vi "insertBundleUnbundle.vi"(2 "error in (no error)":errorcluster, 3 "Controls Cluster":T1(array[cluster]), 4 "action vi path":path) -> (0 "error out":errorcluster, 1 "Indicators":cluster{"Style":u32, "Label.Text":string, i32}[](array[cluster]))   [LabVIEW 2009, in "HGF_VisitorGenerator.lvlib"]
doc: "insert bundle and unbundle node to visitors action.vi"
uses:
  HGF_VisitorGenerator.lvlib
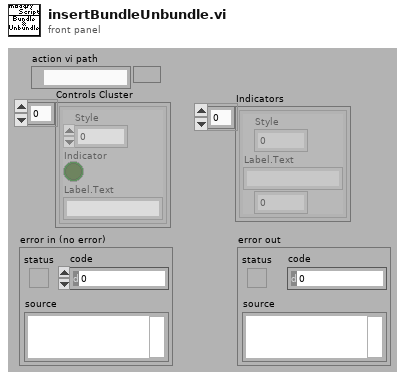
[diagram p1: front panel]
types:
  T1 = cluster{"Style":u32, "Indicator":bool, "Label.Text":string}[]
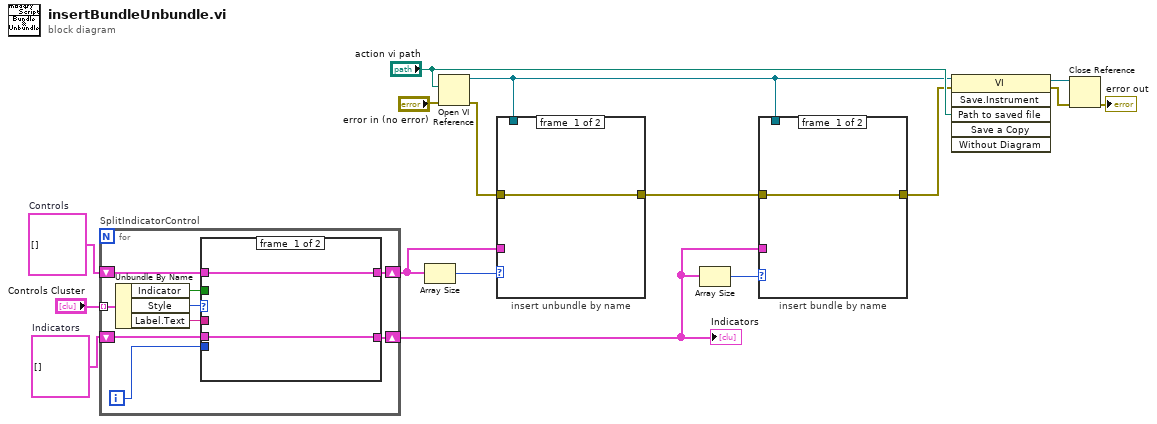
[diagram p0: block diagram]
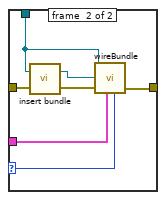
[diagram p2: hidden frame]
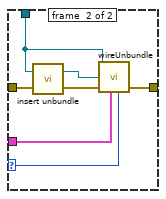
[diagram p3: hidden frame]
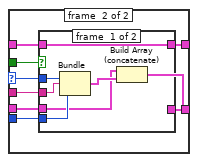
[diagram p4: hidden frame]
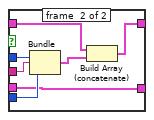
[diagram p5: hidden frame]
diagram:
  w16 = cluster{"Style":u32, "Label.Text":string, i32}[] []  # Indicators
  w15 = cluster{"Style":u32, "Label.Text":string, i32}[] []  # Controls
  n1 = for "SplitIndicatorControl" {
    tunnel: "Controls Cluster" -> [w25] mode=indexing
    shift-right: [w19] -> w2
    shift-left: w15 -> [w21]
    shift-right: [w17] -> w7
    shift-left: w16 -> [w18]
    i -> [w20]
    n2 = Unbundle By Name(w25) -> ("Indicator"=w23:bool, "Style"=w24:u32, "Label.Text"=w22:string)
    n3 = case shown="0" w24 {
      selector: w24 -> [_ w34]
      tunnel: w23 -> [_ w35]
      tunnel: w22 -> [_ w33]
      tunnel: w21 -> [w27 w31]
      tunnel: w20 -> [_ w32]
      tunnel: [w27 w30] -> w19
      tunnel: w18 -> [w26 w29]
      tunnel: [w26 w28] -> w17
      frame #0 {
      }
      frame #1 {
        n4 = case shown="False" w35 {
          tunnel: w34 -> [w42 w47]
          tunnel: w33 -> [w41 w46]
          tunnel: w32 -> [w40 w45]
          tunnel: w31 -> [w38 w49]
          tunnel: [w38 w48] -> w30
          tunnel: w29 -> [w37 w43]
          tunnel: [w36 w43] -> w28
          frame #0 {
            n5 = Bundle("Style"=w42, "Label.Text"=w41, w40) -> (w39:cluster{"Style":u32, "Label.Text":string, i32})  [unwired: 1 in]
            n6 = Build Array (concatenate)(w37, w39) -> (w36:cluster{"Style":u32, "Label.Text":string, i32}[])
          }
          frame #1 {
            n7 = Bundle("Style"=w47, "Label.Text"=w46, w45) -> (w44:cluster{"Style":u32, "Label.Text":string, i32})  [unwired: 1 in]
            n8 = Build Array (concatenate)(w49, w44) -> (w48:cluster{"Style":u32, "Label.Text":string, i32}[])
          }
        }
      }
    }
  }
  "Indicators" <- w7
  n9 = Array Size(array=w2) -> (size(s)=w1:i32)
  n10 = Open VI Reference(vi path="action vi path", error in (no error)="error in (no error)") -> (vi reference=w5:refnum<vi>, error out=w12:errorcluster)  [unwired: 4 in]
  n11 = case "insert unbundle by name" shown="Default" w1 {
    selector: w1 -> [_ w52]
    tunnel: w5 -> [_ w54]
    tunnel: w12 -> [w50 w57]
    tunnel: [w50 w53] -> w4
    tunnel: w2 -> [_ w51]
    frame #0 {
    }
    frame #1 {
      n12 = call "insert unbundle.vi"("error in"=w57, "vi reference"=w54) -> ("error out"=w55:errorcluster, "UnbundleByNameReference"=w56:refnum<vi>)
      n13 = call "wireUnbundle.vi"("vi reference"=w54, "UnbundleByNameReference"=w56, "error in"=w55, "Controls"=w51, "NofInputs"=w52) -> ("error out"=w53:errorcluster)  [unwired: 4 in]
    }
  }
  n14 = Array Size(array=w7) -> (size(s)=w6:i32)
  n15 = case "insert bundle by name" shown="Default" w6 {
    selector: w6 -> [_ w61]
    tunnel: w5 -> [_ w59]
    tunnel: w4 -> [w58 w65]
    tunnel: [w58 w63] -> w3
    tunnel: w7 -> [_ w62]
    frame #0 {
    }
    frame #1 {
      n16 = call "insert bundle.vi"("error in"=w65, "vi reference"=w59) -> ("error out"=w64:errorcluster, "BundleReference"=w60:refnum<vi>)
      n17 = call "wireBundle.vi"("vi reference"=w59, "BundleReference"=w60, "error in"=w64, "Controls"=w62, "NofOutputs"=w61) -> ("error out"=w63:errorcluster)  [unwired: 4 in]
    }
  }
  n18 = invoke class="VI" method="Save.Instrument"(reference=w5, error in=w3, "Path to saved file"="action vi path") -> (reference out=w10:refnum<vi>, error out=w9:errorcluster)  [unwired: 3 in, 4 out]
  n19 = Close Reference(reference=w10, error in (no error)=w9) -> (error out=→"error out":errorcluster)
